vi "Pressure.vi"(8 "error in (no error)":errorcluster, 10 "Pressure":i16, 11 "VISA resource name":refnum<visa-resource-name>) -> (0 "error out":errorcluster, 3 "VISA resource name out":refnum<visa-resource-name>)   [LabVIEW 2021, in "Dispenser.lvclass"]
uses:
  Dispenser.lvclass
  Drivers/EFD Ultimus V/EFD Ultimus V.lvlib
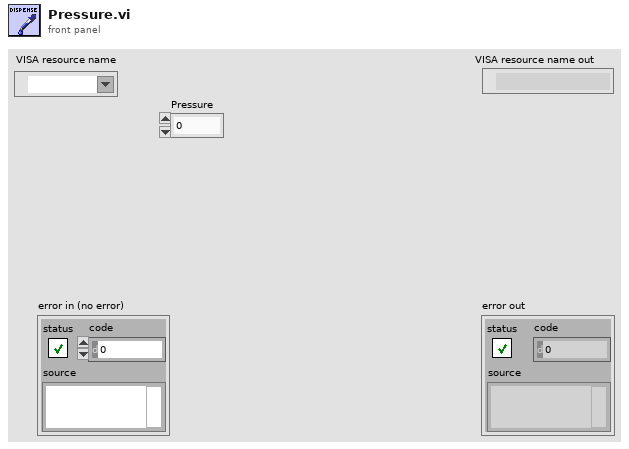
[diagram p1: front panel]
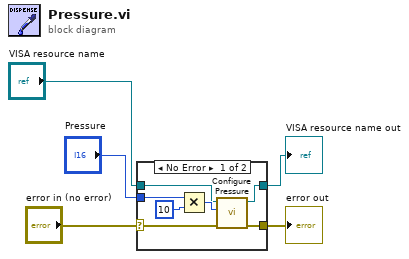
[diagram p0: block diagram]
diagram:
  n1 = case shown="No Error" "error in (no error)" {
    selector: "error in (no error)" -> [w7 w14]
    tunnel: [w6 w14] -> w4
    tunnel: "Pressure" -> [w11 _]
    tunnel: "VISA resource name" -> [w9 w13]
    tunnel: [w8 w13] -> w1
    frame No Error {
      n2 = Multiply(x=w11, y=i16 10) -> (x*y=w10:i16)
      n3 = call "Configure Pressure.vi"("error in (no error)"=w7, "Pressure Setting (0000)"=w10, "VISA resource name"=w9) -> ("error out"=w6:errorcluster, "VISA resource name out"=w8:refnum<visa-resource-name>)  [unwired: 7 in]
    }
    frame Error {
    }
  }
  "error out" <- w4
  "VISA resource name out" <- w1
